vi "Esophageal_CastImage.vi"(5 "X Resolution":i32, 7 "Y Resolution":i32, 8 "error in (no error)":errorcluster, 11 "Image In":T1) -> (0 "error out":errorcluster)   [LabVIEW 2021]
uses:
  <vilib>/vision/Image Controls.llb/IMAQ Image.ctl
  <vilib>/vision/NI_Vision_Development_Module.lvlib
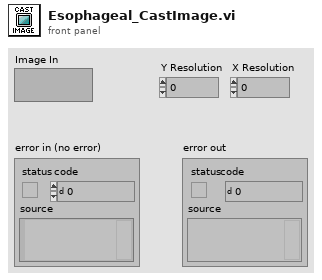
[diagram p1: front panel]
types:
  T1 = typedef "IMAQ Image.ctl" = refnum<image>
  T2 = typedef "Image Type" = u32
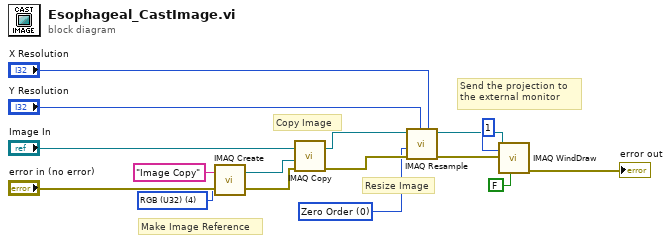
[diagram p0: block diagram]
diagram:
  w9 = u32 0 items=["Zero Order", "Bi-Linear", "Quadratic", "Cubic Spline"] ("Interpolation Type")
  w7 = T2 4 items=["Grayscale (U8)", "Grayscale (I16)", "Grayscale (SGL)", "Complex (CSG)", "RGB (U32)", "HSL (U32)", "RGB (U64)", "Grayscale (U16)"] ("Image Type")
  # "Send the projection to \nthe external monitor"
  # "Make Image Reference"
  # "Resize Image"
  # "Copy Image"
  n1 = call "IMAQ Create"("Image Name"="Image Copy", "Image Type"=w7, "error in (no error)"="error in (no error)") -> ("New Image"=w8:T1, "error out"=w1:errorcluster)  [unwired: 2 in]
  n2 = call "IMAQ Copy"("error in (no error)"=w1, "Image Dst"=w8, "Image Src"="Image In") -> ("error out"=w10:errorcluster, "Image Dst Out"=w11:T1)  [unwired: 3 in]
  n3 = call "IMAQ Resample"("X Resolution"="X Resolution", "Y Resolution"="Y Resolution", "error in (no error)"=w10, "Interpolation Type"=w9, "Image Src"=w11) -> ("error out"=w2:errorcluster, "Image Dst Out"=w3:T1)  [unwired: 5 in]
  n4 = call "IMAQ WindDraw"("Resize to Image Size? (Y)"=FALSE, "Window Number (0...15)"=1, "error in (no error)"=w2, "Image"=w3) -> ("error out"=→"error out":errorcluster)  [unwired: 6 in, 1 out]
